vi "get_device_name.vi"(8 "error in":errorcluster, 11 "VISA resource name in":refnum<visa-resource-name>="COM1") -> (0 "error out":errorcluster, 2 "Device name":string, 3 "VISA resource name out":refnum<visa-resource-name>)   [LabVIEW 2020]
panel:
  in  "Read count":u32
  out "command":string
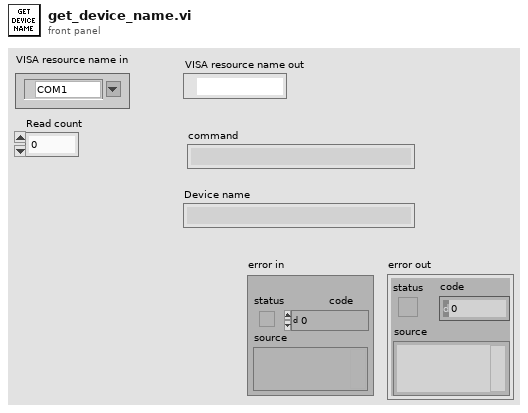
[diagram p1: front panel]
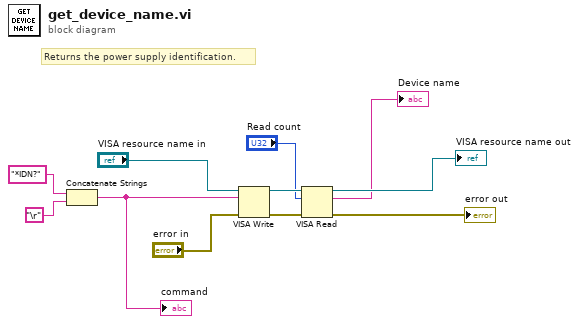
[diagram p0: block diagram]
diagram:
  # "Returns the power supply identification."
  n1 = Concatenate Strings("*IDN?" ("string"), "\r") -> (w8:string)
  "command" <- w8
  n2 = VISA Write(VISA resource name="VISA resource name in", write buffer=w8, error in (no error)="error in") -> (VISA resource name out=w6:refnum<visa-resource-name>, error out=w5:errorcluster)  [unwired: 1 out]
  n3 = VISA Read(VISA resource name=w6, byte count="Read count", error in (no error)=w5) -> (VISA resource name out=→"VISA resource name out":refnum<visa-resource-name>, read buffer=→"Device name":string, error out=→"error out":errorcluster)  [unwired: 1 out]
